vi "Set-speed.vi"(8 "error in (no error)":errorcluster, 10 "Speed":dbl caption="Speed [unit/s]", 11 "Motor in":refnum<class "Motor.lvclass">) -> (0 "error out":errorcluster, 3 "Motor out":refnum<class "Motor.lvclass">)   [LabVIEW 2013, in "PowderDeposition.lvlib" / "Motor.lvclass"]
uses:
  Motor.lvclass
  Motor.lvclass/Motor.ctl
  Main/Custom-errors.ctl
  Main/PD-Main.lvclass
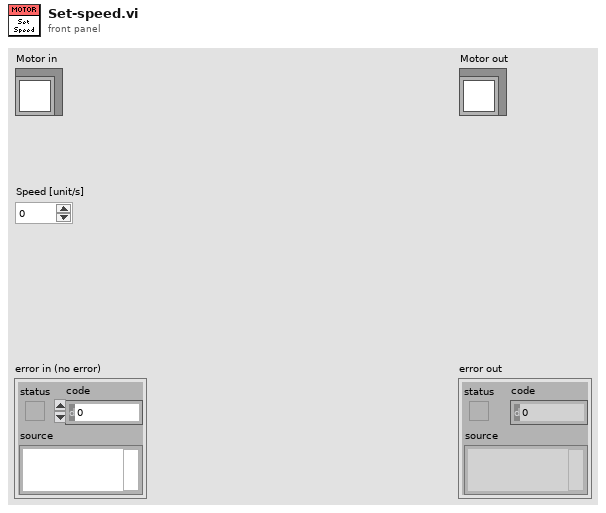
[diagram p1: front panel]
types:
  T1 = typedef "PowderDeposition.lvlib/PD-Main.lvclass/Custom-errors.ctl" = enum16{"Not implemented", "Command not recognized", "Invalid input", "Timeout", "Load file failed", "Action failed", "Action invalid", "Motor inactive", "Not in range", "Unsafe state"}
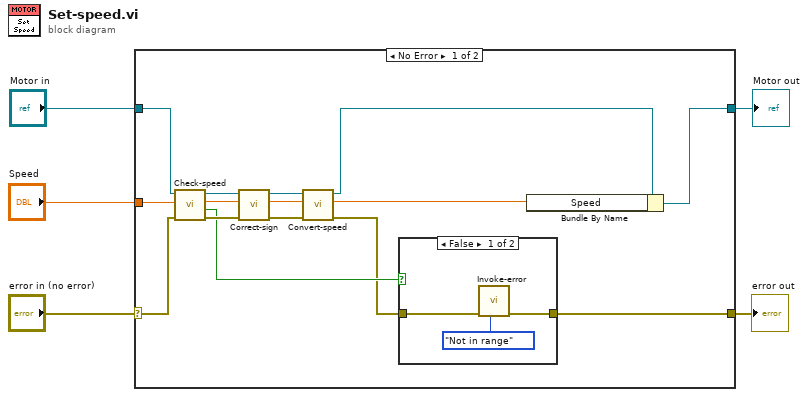
[diagram p0: block diagram]
diagram:
  n1 = case shown="No Error" "error in (no error)" {
    selector: "error in (no error)" -> [w9 w26]
    tunnel: [w6 w26] -> w4
    tunnel: [w20 w25] -> w2
    tunnel: "Motor in" -> [w15 w25]
    tunnel: "Speed" -> [w19 _]
    frame No Error {
      n2 = call-dynamic "Check-speed.vi"("error in (no error)"=w9, "Speed in"=w19, "Motor in"=w15) -> ("error out"=w11:errorcluster, "In range?"=w8:bool, "Speed out"=w18:dbl, "Motor out"=w13:refnum<class "Motor.lvclass">)  [unwired: 5 in]
      n3 = call-dynamic "Correct-sign.vi"("error in (no error)"=w11, "Value in"=w18, "Motor in"=w13) -> ("error out"=w10:errorcluster, "Value out"=w17:dbl, "Motor out"=w12:refnum<class "Motor.lvclass">)  [unwired: 6 in]
      n4 = call-dynamic "Convert-speed.vi"("error in (no error)"=w10, "Speed in"=w17, "Motor in"=w12) -> ("error out"=w7:errorcluster, "Speed out"=w16:dbl, "Motor out"=w14:refnum<class "Motor.lvclass">)  [unwired: 6 in]
      n5 = case shown="False" w8 {
        tunnel: w7 -> [w23 w24]
        tunnel: [w22 w24] -> w6
        frame False {
          n6 = call "Invoke-error.vi"("Error"=Custom-errors."Not in range", "error in (no error)"=w23) -> ("error out"=w22:errorcluster)  [unwired: 9 in]
        }
        frame True {
        }
      }
      n7 = Bundle By Name(cluster=w14, "Speed"=w16) -> (w20:refnum<class "Motor.lvclass">)
    }
    frame Error {
    }
  }
  "error out" <- w4
  "Motor out" <- w2
